vi "VO Channel Config.vi"(8 "error in (no error)":errorcluster, 11 "Node Ptr":T2 format="%.0x") -> (0 "error out":errorcluster)   [LabVIEW 2011, in "Simulated Thermocouple Custom Device.lvlib"]
uses:
  Simulated Thermocouple Custom Device.lvlib
  <vilib>/NI Veristand/Custom Device API/Custom Device Item Ref.ctl
  VO Channel Config Data.ctl
  <vilib>/NI Veristand/Custom Device API/Get Item Property (Variant).vi
  <vilib>/NI Veristand/Custom Device API/Get Item Property (String).vi
  <vilib>/NI Veristand/Custom Device API/Set Item Property (Variant).vi
  <vilib>/NI Veristand/Custom Device API/Set Item Property (String).vi
  <vilib>/regexp/Match Regular Expression.xnode
  <vilib>/NI Veristand/Custom Device API/Custom Device API.lvlib
panel:
  in  "Units":string="V"
  out "Address":string
  in  "Physical Channel":u16(ring) items=["0", "1", "2", "3", "4", "5", "6", "7", "8", "9", "10", "11", "12", "13", "14", "15", "16", "17", "18", "19", "20", "21", "22", "23", "24", "25", "26", "27", "28", "29", "30", "31"]
  in  "Header 3":cluster{"Section Name":string}={"Section Name"="Physical Channel"}
  in  "VO Channel Config":T1={"Initial Value"=0.0, "Range Min"=-10.0, "Range Max"=10.0} {"Range Max" min=-10.0 max=10.0; "Range Min" min=-10.0 max=10.0}
  in  "Header 2":cluster{"Section Name":string}={"Section Name"="Voltage Channel Settings"}
  in  "Header":cluster{"Section Name":string}={"Section Name"="Voltage Channel Specification"}
  in  "Description":string="This page allows you to modify the settings for the physical channel listed at the bottom of this page.  Use the Physical Channel selector to change the hardware resource associated with this Veristand channel."
  in  "Name":string
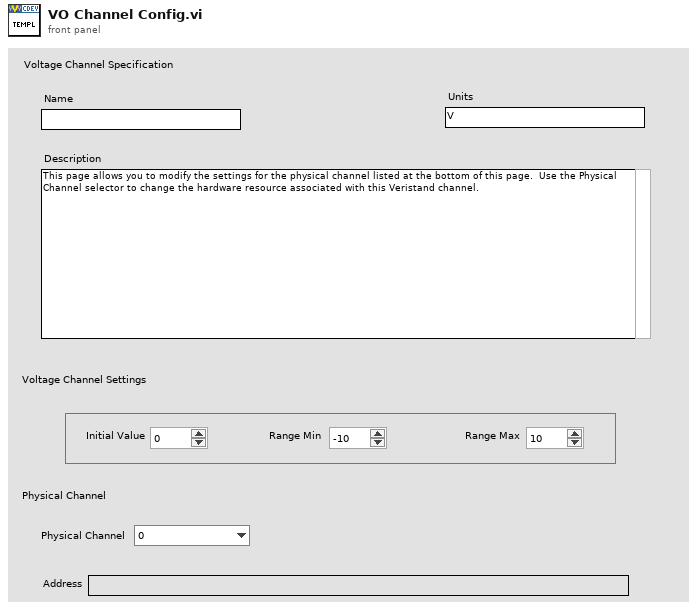
[diagram p1: front panel]
types:
  T1 = typedef "Simulated Thermocouple Custom Device.lvlib/VO Channel Config Data.ctl" = cluster{"Initial Value":dbl, "Range Min":dbl, "Range Max":dbl}
  T2 = typedef "Custom Device API.lvlib/Custom Device Item Ref.ctl" = u64
  T3 = typedef "Custom Device API.lvlib/Custom Device Item Info.ctl" = cluster{"Name":string, "Is Channel":bool, "GUID":string}
  T4 = typedef "Custom Device API.lvlib/Custom Device Commands.ctl" = enum16{"Default", "Item renamed", "Shutdown", "Dynamic button pressed"}
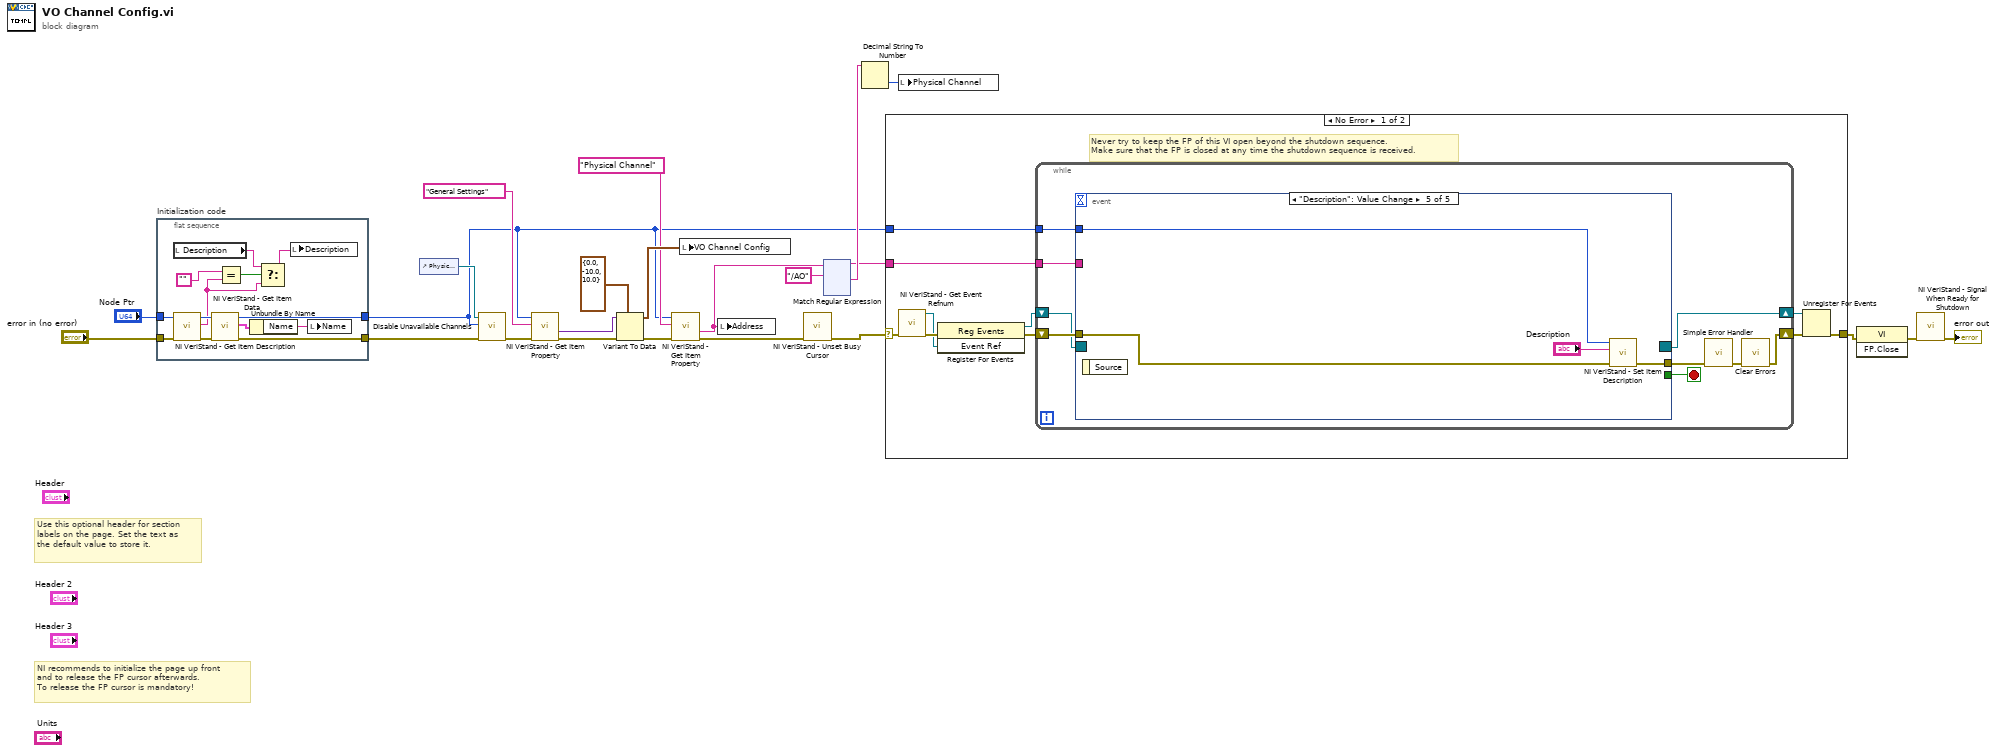
[diagram p0: block diagram]
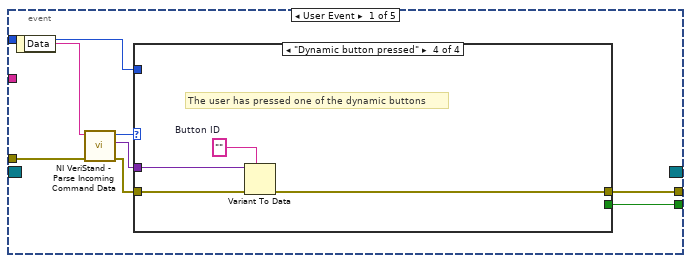
[diagram p2: hidden frame]
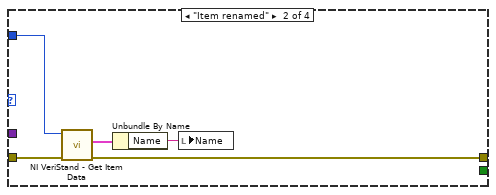
[diagram p4: hidden frame]
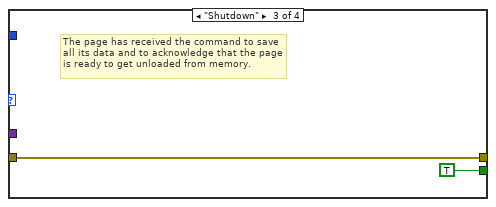
[diagram p5: hidden frame]
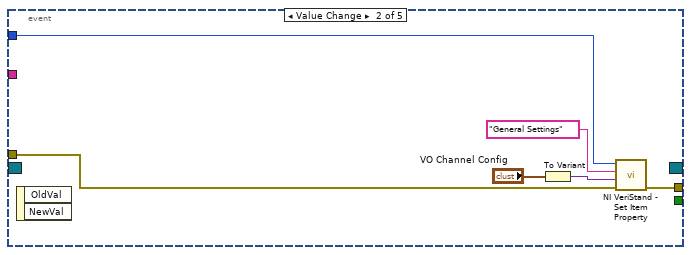
[diagram p6: hidden frame]
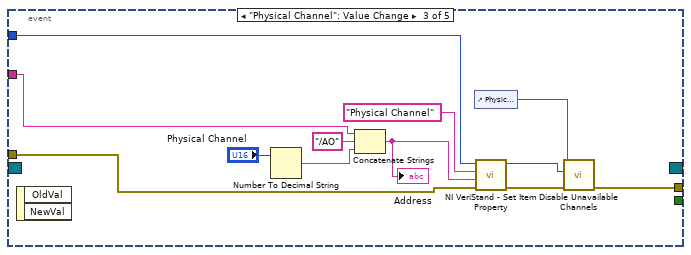
[diagram p7: hidden frame]
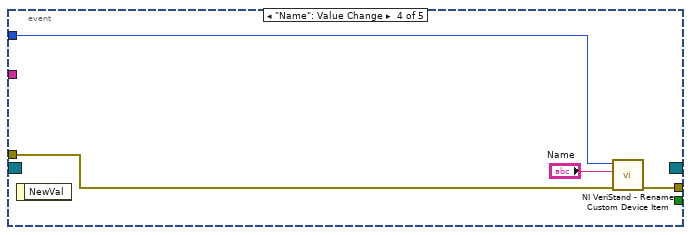
[diagram p8: hidden frame]
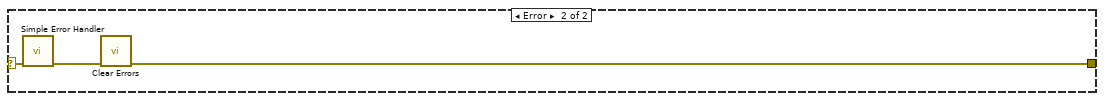
[diagram p9: hidden frame]
diagram:
  # "Use this optional header for section labels on the page. Set the text as the default value to store it."
  # "NI recommends to initialize the page up front\nand to release the FP cursor afterwards.\nTo release the FP cursor is mandatory!"
  n1 = flat-sequence "Initialization code" {
    tunnel: "error in (no error)" -> [w34]
    tunnel: "Node Ptr" -> [w33]
    tunnel: [w29] -> w17
    tunnel: [w36] -> w1
    frame #0 {
      n2 = local read "Description"() -> (w26:string)
      n3 = call <vilib>:"NI VeriStand - Get Item Description.vi"("error in (no error)"=w34, "Item Ref in"=w33) -> ("error out"=w32:errorcluster, "Description"=w24:string, "Item Ref out"=w35:T2)  [unwired: 7 out]
      n4 = call <vilib>:"NI VeriStand - Get Item Data.vi"("error in (no error)"=w32, "Item Ref in"=w35) -> ("error out"=w29:errorcluster, "Item Info"=w31:T3, "Item Ref out"=w36:T2)  [unwired: 7 out]
      n5 = Equal?(x="", y=w24) -> (x = y?=w27:bool)
      n6 = Unbundle By Name(w31) -> ("Name"=w30:string)
      n7 = Select(t=w26, s=w27, f=w24) -> (s? t:f=w25:string)
      n8 = local write "Description"(w25) -> ()
      n9 = local write "Name"(w30) -> ()
    }
  }
  n10 = control-ref of="Physical Channel"() -> (w16:refnum<vi>)
  n11 = call "Disable Unavailable Channels.vi"("error in (no error)"=w17, "Item Ref out"=w1, "Ring in"=w16) -> ("error out"=w15:errorcluster)  [unwired: 8 in]
  n12 = call-poly <vilib>:"NI VeriStand - Get Item Property.vi"("error in (no error)"=w15, "Property Name"="General Settings", "Item Ref in"=w1) -> ("error out"=w2:errorcluster, "Value"=w4:variant)  [unwired: 5 in, 2 out]
  n13 = Variant To Data(error in=w2, type=T1 {"Initial Value"=0.0, "Range Min"=-10.0, "Range Max"=10.0} ("VO Channel Config"), Variant=w4) -> (data=w13:T1, error out=w12:errorcluster)
  n14 = call-poly <vilib>:"NI VeriStand - Get Item Property.vi"("error in (no error)"=w12, "Property Name"="Physical Channel", "Item Ref in"=w1) -> ("error out"=w7:errorcluster, "Value"=w11:string)  [unwired: 5 in, 2 out]
  n15 = local write "VO Channel Config"(w13) -> ()
  n16 = local write "Address"(w11) -> ()
  n17 = call <vilib>:"NI VeriStand - Unset Busy Cursor.vi"("error in (no error)"=w7) -> ("error out"=w19:errorcluster)  [unwired: 10 out]
  n18 = xnode "Match Regular Expression"("input string"=w11, "regular expression"="/AO") -> ("before match"=w6:string, "after match"=w9:string)  [unwired: 4 in, 3 out]
  n19 = Decimal String To Number(string=w9) -> (number=w8:i32)  [unwired: 2 in, 1 out]
  n20 = case shown="No Error" w19 {
    selector: w19 -> [w38 w104]
    tunnel: [w43 w102] -> w23
    tunnel: w1 -> [w39 _]
    tunnel: w6 -> [w37 _]
    frame No Error {
      # "Never try to keep the FP of this VI open beyond the shutdown sequence.\nMake sure that the FP is closed at any time the shutdown sequence is received."
      n21 = call <vilib>:"NI VeriStand - Get Event Refnum.vi"("error in (no error)"=w38) -> ("error out"=w46:errorcluster, "Event Ref"=w42:refnum<user-event>)  [unwired: 9 out]
      n22 = register-events(error in=w46, w42) -> (reference out=w40:refnum<event-registration>, error out=w41:errorcluster)  [unwired: 1 in]
      n23 = while {
        tunnel: w39 -> [w51]
        shift-right: [w48] -> w44
        shift-left: w41 -> [w54]
        shift-right: [w55] -> w45
        shift-left: w40 -> [w53]
        tunnel: w37 -> [w47]
        stop <- w52 stop-if-true
        n24 = event shown="[4] \"Description\": Value Change" {
          selector: w53 -> [_ _ _ _ _]
          dyn-events: [_ _ _ _ _] -> w55
          timeout: _ -> [_ _ _ _ _]
          tunnel: w54 -> [w63 w77 w87 w97 w100]
          tunnel: [w59 _ _ _ _] -> w52
          tunnel: [w58 w76 w82 w96 w99] -> w50
          tunnel: w51 -> [w57 w79 w93 w95 w101]
          tunnel: w47 -> [_ _ w91 _ _]
          event User Event {
            n25 = event-data() -> ("Data"=w62:string)  [unwired: 1 out]
            n26 = call <vilib>:"NI VeriStand - Parse Incoming Command Data.vi"("error in (no error)"=w63, "Incoming data"=w62) -> ("error out"=w61:errorcluster, "Outgoing data"=w56:variant, "Action"=w60:T4)  [unwired: 7 out]
            n27 = case shown="\"Dynamic button pressed\"" w60 {
              tunnel: w61 -> [w64 w69 w70 w75]
              tunnel: [_ _ TRUE _] -> w59
              tunnel: [w64 w66 w70 w72] -> w58
              tunnel: w57 -> [_ w68 _ _]
              tunnel: w56 -> [_ _ _ w74]
              frame "Default", Default {
              }
              frame "Item renamed" {
                n28 = call <vilib>:"NI VeriStand - Get Item Data.vi"("error in (no error)"=w69, "Item Ref in"=w68) -> ("error out"=w66:errorcluster, "Item Info"=w67:T3)  [unwired: 8 out]
                n29 = Unbundle By Name(w67) -> ("Name"=w65:string)
                n30 = local write "Name"(w65) -> ()
              }
              frame "Shutdown" {
                # "The page has received the command to save all its data and to acknowledge that the page is ready to get unloaded from memory."
              }
              frame "Dynamic button pressed" {
                w73 = ""  # Button ID
                # "The user has pressed one of the dynamic buttons"
                n31 = Variant To Data(error in=w75, type=w73, Variant=w74) -> (error out=w72:errorcluster)  [unwired: 1 out]
              }
            }
          }
          event Value Change {
            n32 = event-data() -> ()  [unwired: 3 out]
            n33 = To Variant(anything="VO Channel Config") -> (Variant=w80:variant)
            n34 = call-poly <vilib>:"NI VeriStand - Set Item Property.vi"("error in (no error)"=w77, "Value"=w80, "Property Name"="General Settings", "Item Ref in"=w79) -> ("error out"=w76:errorcluster)  [unwired: 5 in, 2 out]
          }
          event "Physical Channel": Value Change {
            n35 = event-data() -> ()  [unwired: 3 out]
            n36 = Number To Decimal String(number="Physical Channel") -> (decimal integer string=w89:string)  [unwired: 1 in]
            n37 = Concatenate Strings(w91, "/AO" ("regular expression"), w89) -> (w86:string)
            "Address" <- w86
            n38 = control-ref of="Physical Channel"() -> (w84:refnum<vi>)
            n39 = call-poly <vilib>:"NI VeriStand - Set Item Property.vi"("error in (no error)"=w87, "Value"=w86, "Property Name"="Physical Channel", "Item Ref in"=w93) -> ("error out"=w83:errorcluster, "Item Ref out"=w85:T2)  [unwired: 5 in, 1 out]
            n40 = call "Disable Unavailable Channels.vi"("error in (no error)"=w83, "Item Ref out"=w85, "Ring in"=w84) -> ("error out"=w82:errorcluster)  [unwired: 8 in]
          }
          event "Name": Value Change {
            n41 = event-data() -> ()  [unwired: 2 out]
            n42 = call <vilib>:"NI VeriStand - Rename Custom Device Item.vi"("error in (no error)"=w97, "New Name"="Name", "Item Ref in"=w95) -> ("error out"=w96:errorcluster)  [unwired: 8 out]
          }
          event "Description": Value Change {
            n43 = event-data() -> ()  [unwired: 2 out]
            n44 = call <vilib>:"NI VeriStand - Set Item Description.vi"("error in (no error)"=w100, "Description"="Description", "Item Ref in"=w101) -> ("error out"=w99:errorcluster)  [unwired: 8 out]
          }
        }
        n45 = call <vilib>:"Simple Error Handler.vi"("error in (no error)"=w50) -> ("error out"=w49:errorcluster)  [unwired: 1 in, 7 out]
        n46 = call <vilib>:"Clear Errors.vi"("error in (no error)"=w49) -> ("error out"=w48:errorcluster)  [unwired: 6 out]
      }
      n47 = Unregister For Events(event registration refnum=w45, error in=w44) -> (error out=w43:errorcluster)
    }
    frame Error {
      n48 = call <vilib>:"Simple Error Handler.vi"("error in (no error)"=w104) -> ("error out"=w103:errorcluster)  [unwired: 1 in, 7 out]
      n49 = call <vilib>:"Clear Errors.vi"("error in (no error)"=w103) -> ("error out"=w102:errorcluster)  [unwired: 6 out]
    }
  }
  n50 = local write "Physical Channel"(w8) -> ()
  n51 = invoke class="VI" method="FP.Close"(error in=w23) -> (error out=w22:errorcluster)  [unwired: 2 in, 2 out]
  n52 = call <vilib>:"NI VeriStand - Signal When Ready for Shutdown.vi"("error in (no error)"=w22) -> ("error out"=→"error out":errorcluster)  [unwired: 10 out]
